vi "Make.vi"() -> ()   [LabVIEW 2019]
doc: "Quick and dirty makefile."
uses:
  <vilib>/AppBuilder/AB_API_Simple/Build (path).vi
  <vilib>/AppBuilder/AB_API_Simple/NI_App_Builder_API.lvlib
panel:
  out "error out":errorcluster
  out "Currently building":path
  out "Generated files":path[](array[path])
  # "Note: Ensure all projects are closed in memory, then run this VI."
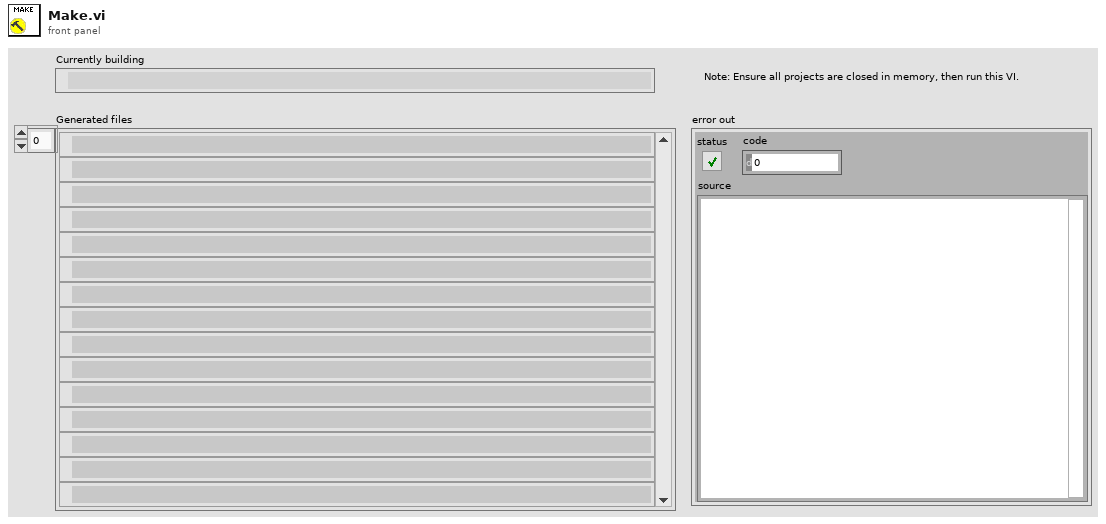
[diagram p1: front panel]
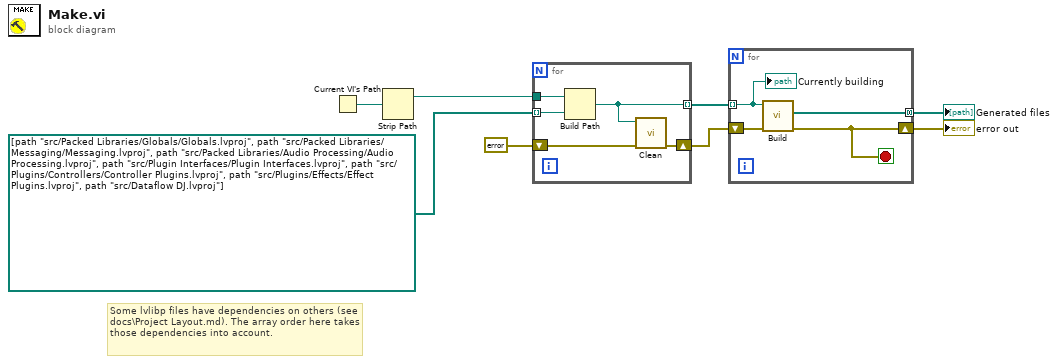
[diagram p0: block diagram]
diagram:
  # "Some lvlibp files have dependencies on others (see docs\\Project Layout.md). The array order here takes those dependencies into account."
  n1 = Current VI's Path() -> (path=w8:path)
  n2 = Strip Path(path=w8) -> (stripped path=w6:path)  [unwired: 1 out]
  n3 = for {
    tunnel: path[] [path "src/Packed Libraries/Globals/Globals.lvproj", path "src/Packed Libraries/Messaging/Messaging.lvproj", path "src/Packed Libraries/Audio Processing/Audio Processing.lvproj", path "src/Plugin Interfaces/Plugin Interfaces.lvproj", path "src/Plugins/Controllers/Controller Plugins.lvproj", path "src/Plugins/Effects/Effect Plugins.lvproj", path "src/Dataflow DJ.lvproj"] -> [w13] mode=indexing
    tunnel: w6 -> [w12]
    tunnel: [w11] -> w3 mode=indexing
    shift-right: [w10] -> w2
    shift-left: errorcluster {"status"=FALSE, "code"=0, "source"=""} ("error out") -> [w9]
    n4 = Build Path(base path=w12, name or relative path=w13) -> (appended path=w11:path)
    n5 = call <vilib>:"Clean.vi"("error in (no error)"=w9, "Path to project"=w11) -> ("error out"=w10:errorcluster)  [unwired: 9 in]
  }
  n6 = for {
    tunnel: [w17] -> w5 mode=concatenating
    tunnel: w3 -> [w16] mode=indexing
    shift-right: [w15] -> w4
    shift-left: w2 -> [w14]
    stop <- w15 stop-if-true
    n7 = call-poly <vilib>:"Build.vi"("error in (no error)"=w14, "Path to project"=w16) -> ("error out"=w15:errorcluster, "Generated files"=w17:path[])  [unwired: 8 in]
    "Currently building" <- w16
  }
  "Generated files" <- w5
  "error out" <- w4
